vi "Data Fetch.vi"(0 "VISA resource name":refnum<visa-resource-name>, 7 "Channel 1-8 (0:Ch1)":u8(ring) items=["Channel 1", "Channel 2", "Channel 3", "Channel 4", "Channel 5", "Channel 6", "Channel 7", "Channel 8 "], 11 "error in (no error)":errorcluster) -> (4 "VISA resource name out":refnum<visa-resource-name>, 6 "Voltage (V)":sgl format="%.4f", 8 "Current (A)":sgl format="%.4f", 10 "Status":bool[](array[boolean]), 15 "error out":errorcluster)   [LabVIEW 2015, in "Chroma ATE 6310.lvlib"]
doc: "This vi returns the real time current and voltage measured at the input of the load module,and shows the real time status of the load module."
uses:
  <instrlib>/Chroma ATE 6310/Chroma ATE 6310.lvlib
panel:
  # "OC                OV                 OP                 RV                OT"
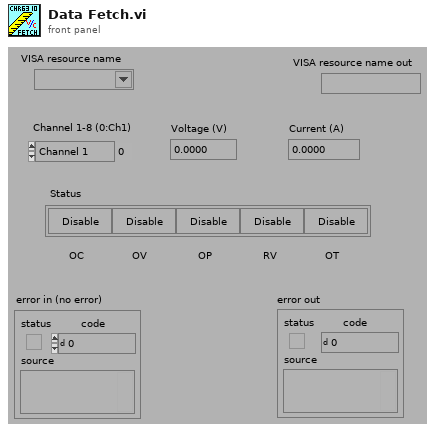
[diagram p1: front panel]
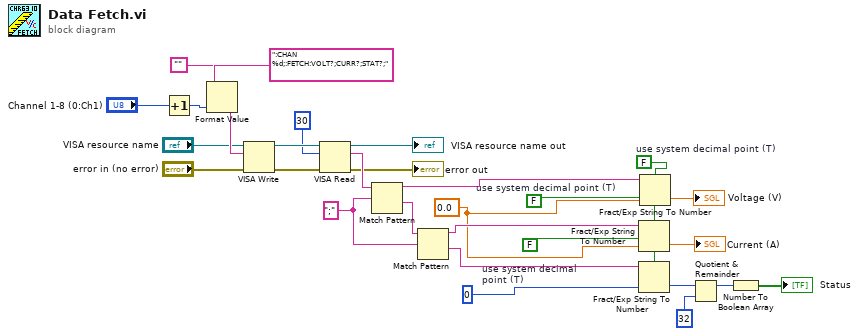
[diagram p0: block diagram]
diagram:
  w1 = FALSE  # use system decimal point (T)
  w2 = FALSE  # use system decimal point (T)
  w3 = FALSE  # use system decimal point (T)
  w5 = sgl 0.0 ("default (0 sgl)")
  w27 = ";"
  n1 = Increment(x="Channel 1-8 (0:Ch1)") -> (x+1=w18:u8)
  n2 = Format Value(string ("")="", format string=":CHAN %d;:FETCH:VOLT?;CURR?;STAT?;", value (0)=w18) -> (output string=w24:string)
  n3 = VISA Write(VISA resource name="VISA resource name", write buffer=w24, error in (no error)="error in (no error)") -> (VISA resource name out=w22:refnum<visa-resource-name>, error out=w23:errorcluster)  [unwired: 1 out]
  n4 = VISA Read(VISA resource name=w22, byte count=u32 30, error in (no error)=w23) -> (VISA resource name out=→"VISA resource name out":refnum<visa-resource-name>, read buffer=w19:string, error out=→"error out":errorcluster)  [unwired: 1 out]
  n5 = Match Pattern(string=w19, regular expression=w27) -> (before substring=w20:string, after substring=w12:string)  [unwired: 1 in, 2 out]
  n6 = Match Pattern(string=w12, regular expression=w27) -> (before substring=w11:string, after substring=w10:string)  [unwired: 1 in, 2 out]
  n7 = Fract/Exp String To Number(use system decimal point (T)=w2, string=w11, default (0 dbl)=w5) -> (number=→"Current (A)":sgl)  [unwired: 1 in, 1 out]
  n8 = Fract/Exp String To Number(use system decimal point (T)=w3, string=w10, default (0 dbl)=0 ("default (0 I32)")) -> (number=w8:i32)  [unwired: 1 in, 1 out]
  n9 = Fract/Exp String To Number(use system decimal point (T)=w1, string=w20, default (0 dbl)=w5) -> (number=→"Voltage (V)":sgl)  [unwired: 1 in, 1 out]
  n10 = Quotient & Remainder(x=w8, y=32) -> (x-y*floor(x/y)=w7:i32)  [unwired: 1 out]
  n11 = Number To Boolean Array(number=w7) -> (Boolean array=→"Status":bool[])
